vi "Data Value Ref to Variant.vi"(8 "error in (no error)":errorcluster, 11 "Data Value Ref":T3) -> (0 "error out":errorcluster, 1 "Type Descriptor":T1[](array[typedef]), 2 "Variant":variant, 3 "Data Value Ref out":T3)   [LabVIEW 2020, in "NI_VS Sequence Execution Interface.lvlib"]
doc: "Translates the data value reference returned by the Get Sequence Return Value VI or a sequence complete event into a LabVIEW variant data type that corresponds to the data type of the sequence return value."
uses:
  <vilib>/NI VeriStand/Execution/SequenceExecutionInterface/NI_VS Sequence Execution Interface.lvlib
  <vilib>/NI VeriStand/Execution/SequenceExecutionInterface/Data Value Ref.ctl
  NationalInstruments.VeriStand.DataTypes
  <vilib>/NI VeriStand/Execution/SequenceExecutionInterface/Type Descriptor Element.ctl
  <vilib>/NI VeriStand/Execution/SequenceExecutionInterface/Data Type.ctl
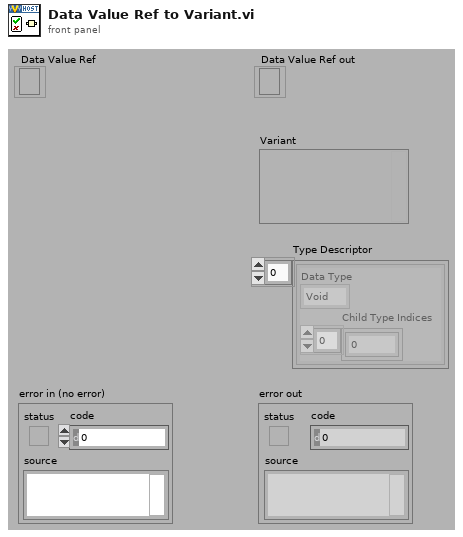
[diagram p1: front panel]
types:
  T1 = typedef "NI_VS Sequence Execution Interface.lvlib/Type Descriptor Element.ctl" = cluster{"Data Type":T2, "Child Type Indices":i32[]}
  T2 = typedef "NI_VS Sequence Execution Interface.lvlib/Data Type.ctl" = enum16{"Void", "Boolean", "Int32", "UInt32", "Int64", "UInt64", "Double", "Array"}
  T3 = typedef "NI_VS Sequence Execution Interface.lvlib/Data Value Ref.ctl" = refnum<k24>
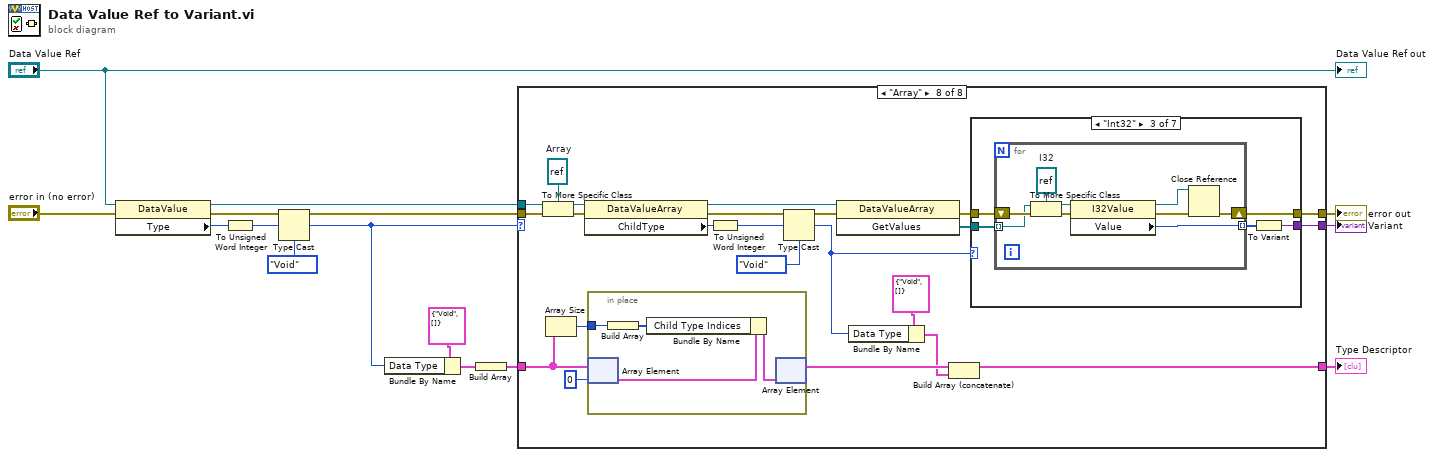
[diagram p0: block diagram]
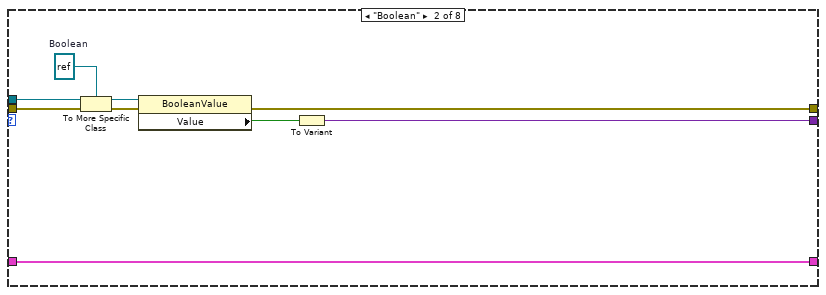
[diagram p3: hidden frame]
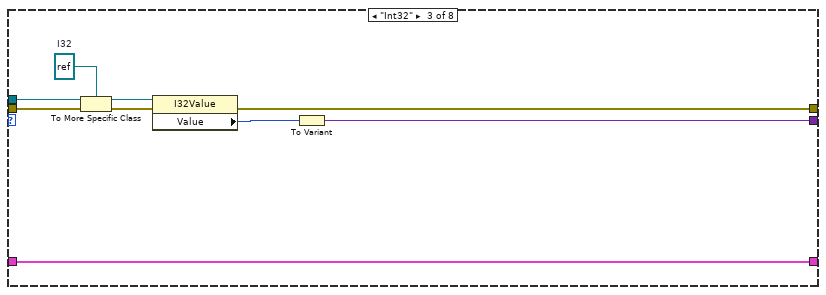
[diagram p4: hidden frame]
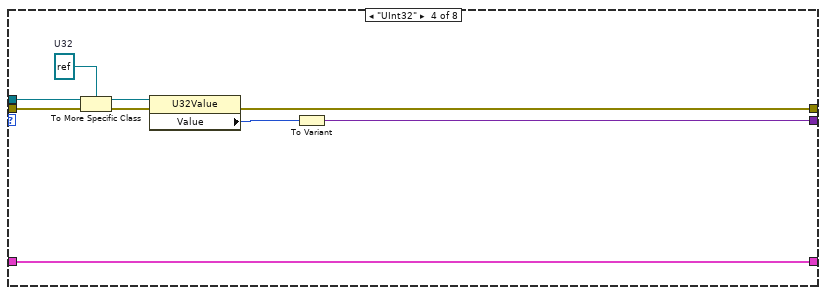
[diagram p5: hidden frame]
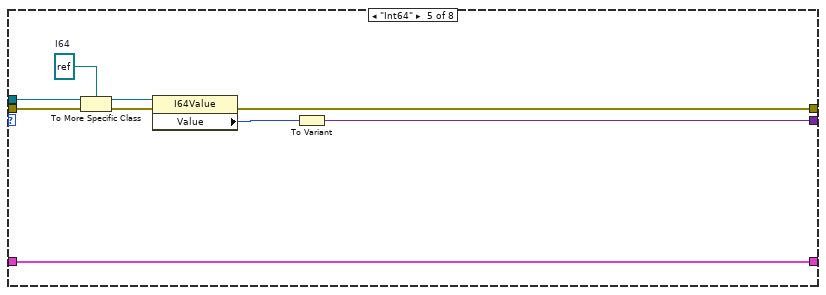
[diagram p6: hidden frame]
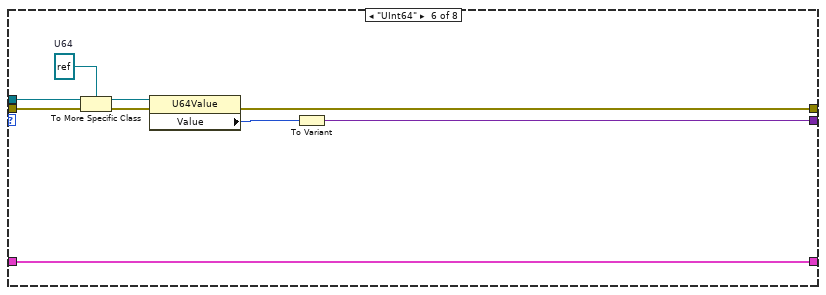
[diagram p7: hidden frame]
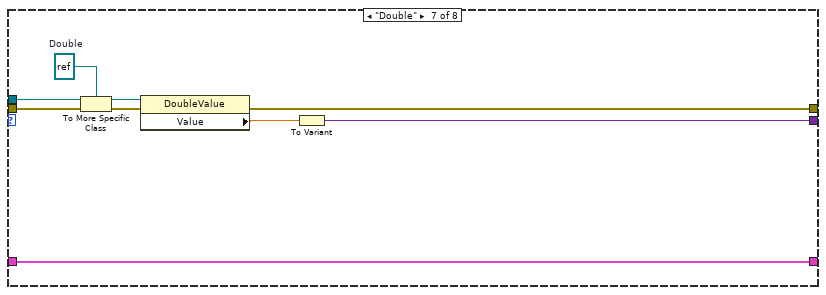
[diagram p8: hidden frame]
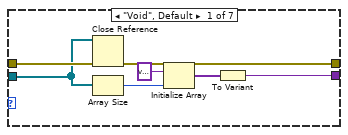
[diagram p9: hidden frame]
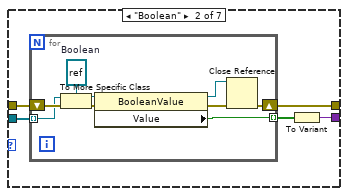
[diagram p10: hidden frame]
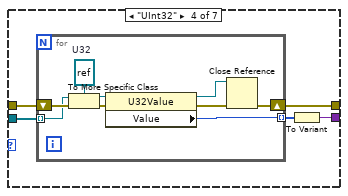
[diagram p11: hidden frame]
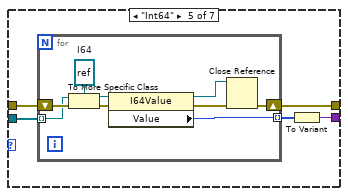
[diagram p12: hidden frame]
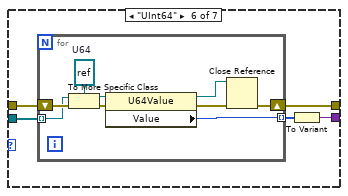
[diagram p13: hidden frame]
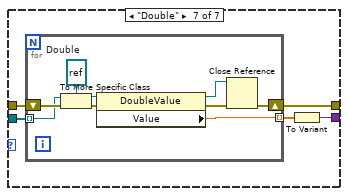
[diagram p14: hidden frame]
diagram:
  n1 = property class="DataValue"(reference="Data Value Ref", error in="error in (no error)") -> (reference out=w9:T3, error out=w10:errorcluster, "Type"=w13:i32)
  n2 = To Unsigned Word Integer(number=w13) -> (unsigned 16bit integer=w12:u16)
  n3 = Type Cast(type=Data_Type."Void" ("Data Type"), x=w12) -> (*(type *) &x=w4:T2)
  n4 = Bundle By Name(cluster=T1 {"Data Type"=enum."Void", "Child Type Indices"=[]} ("Type Descriptor Element"), "Data Type"=w4) -> (w3:T1)
  n5 = Build Array(w3) -> (w2:T1[])
  n6 = case shown="\"Array\"" w4 {
    tunnel: w10 -> [w16 w24 w33 w42 w51 w60 w69 w90]
    tunnel: w9 -> [_ w25 w34 w43 w52 w61 w70 w91]
    tunnel: [_ w18 w27 w36 w45 w54 w63 w79] -> w8
    tunnel: [w16 w20 w29 w38 w47 w56 w65 w78] -> w7
    tunnel: [w15 w17 w26 w35 w44 w53 w62 w74] -> w1
    tunnel: w2 -> [w15 w17 w26 w35 w44 w53 w62 w72]
    frame "Void", Default {
    }
    frame "Boolean" {
      w23 = refnum<k24> refnum  # Boolean
      n7 = To More Specific Class(target class=w23, reference=w25, error in=w24) -> (specific class reference=w22:refnum<k24>, error out=w21:errorcluster)
      n8 = property class="BooleanValue"(reference=w22, error in=w21) -> (error out=w20:errorcluster, "Value"=w19:bool)  [unwired: 1 out]
      n9 = To Variant(anything=w19) -> (Variant=w18:variant)
    }
    frame "Int32" {
      w32 = refnum<k24> refnum  # I32
      n10 = To More Specific Class(target class=w32, reference=w34, error in=w33) -> (specific class reference=w31:refnum<k24>, error out=w30:errorcluster)
      n11 = property class="I32Value"(reference=w31, error in=w30) -> (error out=w29:errorcluster, "Value"=w28:i32)  [unwired: 1 out]
      n12 = To Variant(anything=w28) -> (Variant=w27:variant)
    }
    frame "UInt32" {
      w41 = refnum<k24> refnum  # U32
      n13 = To More Specific Class(target class=w41, reference=w43, error in=w42) -> (specific class reference=w40:refnum<k24>, error out=w39:errorcluster)
      n14 = property class="U32Value"(reference=w40, error in=w39) -> (error out=w38:errorcluster, "Value"=w37:u32)  [unwired: 1 out]
      n15 = To Variant(anything=w37) -> (Variant=w36:variant)
    }
    frame "Int64" {
      w50 = refnum<k24> refnum  # I64
      n16 = To More Specific Class(target class=w50, reference=w52, error in=w51) -> (specific class reference=w49:refnum<k24>, error out=w48:errorcluster)
      n17 = property class="I64Value"(reference=w49, error in=w48) -> (error out=w47:errorcluster, "Value"=w46:i64)  [unwired: 1 out]
      n18 = To Variant(anything=w46) -> (Variant=w45:variant)
    }
    frame "UInt64" {
      w59 = refnum<k24> refnum  # U64
      n19 = To More Specific Class(target class=w59, reference=w61, error in=w60) -> (specific class reference=w58:refnum<k24>, error out=w57:errorcluster)
      n20 = property class="U64Value"(reference=w58, error in=w57) -> (error out=w56:errorcluster, "Value"=w55:u64)  [unwired: 1 out]
      n21 = To Variant(anything=w55) -> (Variant=w54:variant)
    }
    frame "Double" {
      w68 = refnum<k24> refnum  # Double
      n22 = To More Specific Class(target class=w68, reference=w70, error in=w69) -> (specific class reference=w67:refnum<k24>, error out=w66:errorcluster)
      n23 = property class="DoubleValue"(reference=w67, error in=w66) -> (error out=w65:errorcluster, "Value"=w64:dbl)  [unwired: 1 out]
      n24 = To Variant(anything=w64) -> (Variant=w63:variant)
    }
    frame "Array" {
      w89 = refnum<k24> refnum  # Array
      n25 = To More Specific Class(target class=w89, reference=w91, error in=w90) -> (specific class reference=w88:refnum<k24>, error out=w87:errorcluster)
      n26 = Array Size(array=w72) -> (size(s)=w71:i32)
      n27 = property class="DataValueArray"(reference=w88, error in=w87) -> (reference out=w83:refnum<k24>, error out=w82:errorcluster, "ChildType"=w84:i32)
      n28 = in-place {
        in-place-border: w71 -> [w94]
        n29 = in-place-array #1(w72, 0) -> (w96:T1)
        n30 = Build Array(w94) -> (w93:i32[])
        n31 = Bundle By Name(cluster=w96, "Child Type Indices"=w93) -> (w95:T1)
        n32 = in-place-array #1(w95) -> (w92:T1[])  [unwired: 1 out]
      }
      n33 = To Unsigned Word Integer(number=w84) -> (unsigned 16bit integer=w85:u16)
      n34 = Type Cast(type=Data_Type."Void" ("Data Type"), x=w85) -> (*(type *) &x=w76:T2)
      n35 = invoke class="DataValueArray" method="GetValues"(reference=w83, error in=w82) -> (error out=w80:errorcluster, "GetValues"=w81:refnum<k24>[])  [unwired: 1 in, 1 out]
      n36 = Bundle By Name(cluster=T1 {"Data Type"=enum."Void", "Child Type Indices"=[]} ("Type Descriptor Element"), "Data Type"=w76) -> (w75:T1)
      n37 = Build Array (concatenate)(w92, w75) -> (w74:T1[])
      n38 = case shown="\"Int32\"" w76 {
        tunnel: w81 -> [w101 w108 w122 w136 w150 w164 w178]
        tunnel: w80 -> [w103 w107 w121 w135 w149 w163 w177]
        tunnel: [w97 w106 w120 w134 w148 w162 w176] -> w78
        tunnel: [w98 w104 w118 w132 w146 w160 w174] -> w79
        frame "Void", Default {
          n39 = Close Reference(reference=w101, error in (no error)=w103) -> (error out=w97:errorcluster)
          n40 = Array Size(array=w101) -> (size(s)=w100:i32)
          n41 = Initialize Array(variant ("Variant"), w100) -> (w99:variant[])
          n42 = To Variant(anything=w99) -> (Variant=w98:variant)
        }
        frame "Boolean" {
          n43 = for {
            tunnel: w108 -> [w113] mode=indexing
            shift-right: [w110] -> w106
            shift-left: w107 -> [w117]
            tunnel: [w109] -> w105 mode=indexing
            w116 = refnum<k24> refnum  # Boolean
            n44 = To More Specific Class(target class=w116, reference=w113, error in=w117) -> (specific class reference=w115:refnum<k24>, error out=w114:errorcluster)
            n45 = property class="BooleanValue"(reference=w115, error in=w114) -> (reference out=w112:refnum<k24>, error out=w111:errorcluster, "Value"=w109:bool)
            n46 = Close Reference(reference=w112, error in (no error)=w111) -> (error out=w110:errorcluster)
          }
          n47 = To Variant(anything=w105) -> (Variant=w104:variant)
        }
        frame "Int32" {
          n48 = for {
            tunnel: w122 -> [w127] mode=indexing
            shift-right: [w124] -> w120
            shift-left: w121 -> [w131]
            tunnel: [w123] -> w119 mode=indexing
            w130 = refnum<k24> refnum  # I32
            n49 = To More Specific Class(target class=w130, reference=w127, error in=w131) -> (specific class reference=w129:refnum<k24>, error out=w128:errorcluster)
            n50 = property class="I32Value"(reference=w129, error in=w128) -> (reference out=w126:refnum<k24>, error out=w125:errorcluster, "Value"=w123:i32)
            n51 = Close Reference(reference=w126, error in (no error)=w125) -> (error out=w124:errorcluster)
          }
          n52 = To Variant(anything=w119) -> (Variant=w118:variant)
        }
        frame "UInt32" {
          n53 = for {
            tunnel: w136 -> [w141] mode=indexing
            shift-right: [w138] -> w134
            shift-left: w135 -> [w145]
            tunnel: [w137] -> w133 mode=indexing
            w144 = refnum<k24> refnum  # U32
            n54 = To More Specific Class(target class=w144, reference=w141, error in=w145) -> (specific class reference=w143:refnum<k24>, error out=w142:errorcluster)
            n55 = property class="U32Value"(reference=w143, error in=w142) -> (reference out=w140:refnum<k24>, error out=w139:errorcluster, "Value"=w137:u32)
            n56 = Close Reference(reference=w140, error in (no error)=w139) -> (error out=w138:errorcluster)
          }
          n57 = To Variant(anything=w133) -> (Variant=w132:variant)
        }
        frame "Int64" {
          n58 = for {
            tunnel: w150 -> [w155] mode=indexing
            shift-right: [w152] -> w148
            shift-left: w149 -> [w159]
            tunnel: [w151] -> w147 mode=indexing
            w158 = refnum<k24> refnum  # I64
            n59 = To More Specific Class(target class=w158, reference=w155, error in=w159) -> (specific class reference=w157:refnum<k24>, error out=w156:errorcluster)
            n60 = property class="I64Value"(reference=w157, error in=w156) -> (reference out=w154:refnum<k24>, error out=w153:errorcluster, "Value"=w151:i64)
            n61 = Close Reference(reference=w154, error in (no error)=w153) -> (error out=w152:errorcluster)
          }
          n62 = To Variant(anything=w147) -> (Variant=w146:variant)
        }
        frame "UInt64" {
          n63 = for {
            tunnel: w164 -> [w169] mode=indexing
            shift-right: [w166] -> w162
            shift-left: w163 -> [w173]
            tunnel: [w165] -> w161 mode=indexing
            w172 = refnum<k24> refnum  # U64
            n64 = To More Specific Class(target class=w172, reference=w169, error in=w173) -> (specific class reference=w171:refnum<k24>, error out=w170:errorcluster)
            n65 = property class="U64Value"(reference=w171, error in=w170) -> (reference out=w168:refnum<k24>, error out=w167:errorcluster, "Value"=w165:u64)
            n66 = Close Reference(reference=w168, error in (no error)=w167) -> (error out=w166:errorcluster)
          }
          n67 = To Variant(anything=w161) -> (Variant=w160:variant)
        }
        frame "Double" {
          n68 = for {
            tunnel: w178 -> [w183] mode=indexing
            shift-right: [w180] -> w176
            shift-left: w177 -> [w187]
            tunnel: [w179] -> w175 mode=indexing
            w186 = refnum<k24> refnum  # Double
            n69 = To More Specific Class(target class=w186, reference=w183, error in=w187) -> (specific class reference=w185:refnum<k24>, error out=w184:errorcluster)
            n70 = property class="DoubleValue"(reference=w185, error in=w184) -> (reference out=w182:refnum<k24>, error out=w181:errorcluster, "Value"=w179:dbl)
            n71 = Close Reference(reference=w182, error in (no error)=w181) -> (error out=w180:errorcluster)
          }
          n72 = To Variant(anything=w175) -> (Variant=w174:variant)
        }
      }
    }
  }
  "error out" <- w7
  "Variant" <- w8
  "Type Descriptor" <- w1
  "Data Value Ref out" <- "Data Value Ref"
